vi "Mouse Move.vi"(7 "Map Model in":refnum<class "Map Model.lvclass">, 8 "error in (no error)":errorcluster, 10 "Position":T1, 11 "Pan in":refnum<class "Pan.lvclass">) -> (0 "error out":errorcluster, 3 "Pan out":refnum<class "Pan.lvclass">, 5 "Map Model out":refnum<class "Map Model.lvclass">)   [LabVIEW 2020, in "Map Model.lvlib" / "Pan.lvclass"]
uses:
  Pan.lvclass
  E:/Project/Labview-Projects/Completed projects/Map Editor/Models/Map Model/Tools/Tool/Tool.lvclass
  <vilib>/Utility/miscctls.llb/LVPoint32TypeDef.ctl
  Map Model/Map Model.lvclass
  Tool/Tool.lvclass/Tool.ctl
  Map Model/Map Model.lvclass/Map Model.ctl
  Undoable Tool/Undoable Tool.lvclass
  Tool/Tool.lvclass
  <vilib>/LabVIEW Icon API/lv_icon/lv_icon.lvlib
panel:
  # "NOTICE -- YOU MUST LEAVE THIS NOTICE IN PLACE.\n\nCopyright (c) 2017, LIANG LIU Shawn.Liu.cn@gmail.com\nAll rights reserved.\n\nRedistribution and use in source and binary forms, with or without modification, are permitted provided that the following conditions are met:\n-Redistributions of source code must retain the above copyright notice, this list of conditions and the following disclaimer.\n-Redistributions in binary form must reproduce the above copyright notice, this list of conditions and the following disclaimer in the documentation and/or other materials provided with the distribution.\n-Neither the name of the eLp nor the names of its contributors may be used to endorse or promote products derived from this software without specific prior written permission.\n\nTHIS SOFTWARE IS PROVIDED BY THE COPYRIGHT HOLDERS AND CONTRIBUTORS \"AS IS\" AND ANY EXPRESS OR IMPLIED WARRANTIES, INCLUDING, BUT NOT LIMITED TO, THE IMPLIED WARRANTIES OF MERCHANTABILITY AND FITNESS FOR A PARTICULAR PURPOSE ARE DISCLAIMED. IN NO EVENT SHALL THE COPYRIGHT HOLDER OR CONTRIBUTORS BE LIABLE FOR ANY DIRECT, INDIRECT, INCIDENTAL, SPECIAL, EXEMPLARY, OR CONSEQUENTIAL DAMAGES (INCLUDING, BUT NOT LIMITED TO, PROCUREMENT OF SUBSTITUTE GOODS OR SERVICES; LOSS OF USE, DATA, OR PROFITS; OR BUSINESS INTERRUPTION) HOWEVER CAUSED AND ON ANY THEORY OF LIABILITY, WHETHER IN CONTRACT, STRICT LIABILITY, OR TORT (INCLUDING NEGLIGENCE OR OTHERWISE) ARISING IN ANY WAY OUT OF THE USE OF THIS SOFTWARE, EVEN IF ADVISED OF THE POSSIBILITY OF SUCH DAMAGE."
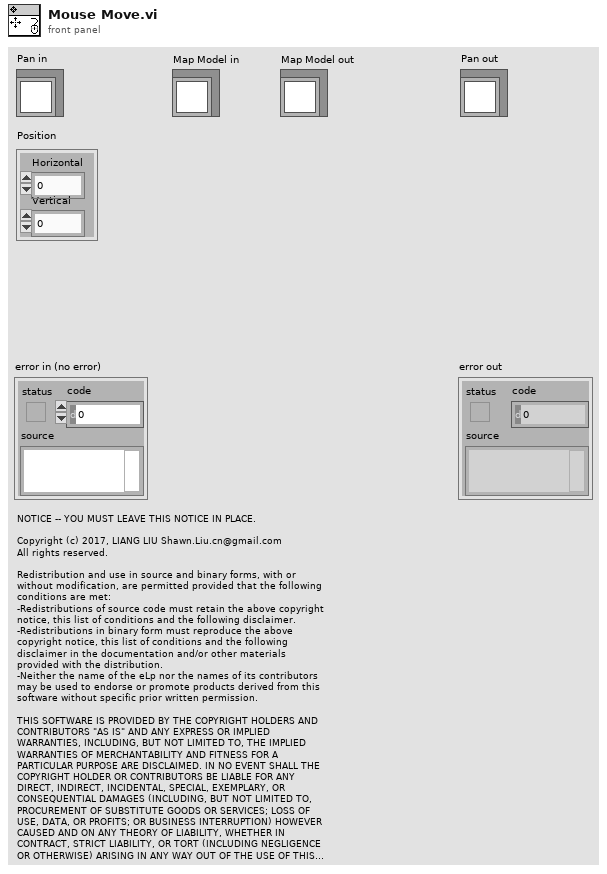
[diagram p1: front panel]
types:
  T1 = typedef "LVPoint32TypeDef.ctl" = cluster{"Horizontal":i32, "Vertical":i32}
  T2 = typedef "imagedata.ctl" = cluster{"image type":i32, "image depth":i32, "image":u8[], "mask":u8[], "colors":u32[], "Rectangle":cluster{"left":i16, "top":i16, "right":i16, "bottom":i16}}
  T3 = cluster{"left":i16, "top":i16, "right":i16, "bottom":i16}
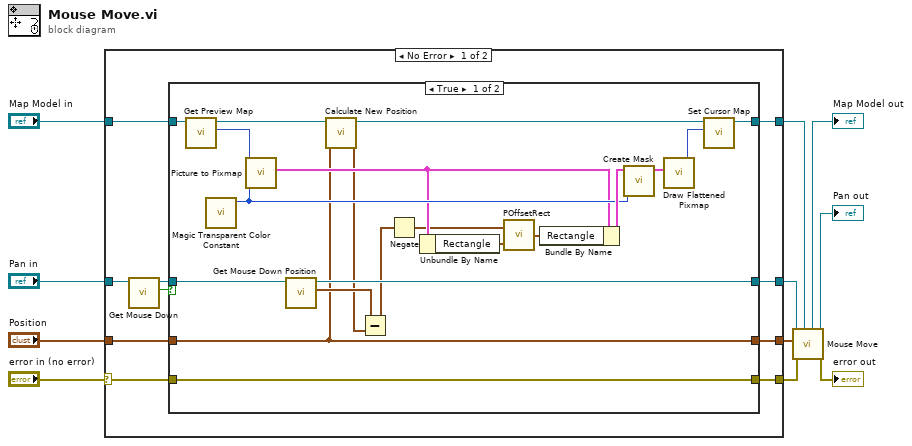
[diagram p0: block diagram]
diagram:
  n1 = case shown="No Error" "error in (no error)" {
    selector: "error in (no error)" -> [w19 w49]
    tunnel: "Map Model in" -> [w21 w48]
    tunnel: "Position" -> [w20 w46]
    tunnel: "Pan in" -> [w18 w47]
    tunnel: [w17 w46] -> w6
    tunnel: [w16 w48] -> w5
    tunnel: [w15 w47] -> w4
    tunnel: [w14 w49] -> w3
    frame No Error {
      n2 = call "Get Mouse Down.vi"("Tool in"=w18) -> ("Mouse Down"=w12:bool, "Tool out"=w13:refnum<class "Pan.lvclass">)  [unwired: 9 in]
      n3 = case shown="True" w12 {
        tunnel: w13 -> [w41 w45]
        tunnel: w21 -> [w39 w43]
        tunnel: [w22 w43] -> w16
        tunnel: [w40 w45] -> w15
        tunnel: w20 -> [w24 w42]
        tunnel: [w24 w42] -> w17
        tunnel: w19 -> [w38 w44]
        tunnel: [w38 w44] -> w14
        frame True {
          n4 = call "Get Preview Map.vi"("Map Model in"=w39) -> ("Preview Map"=w27:picture, "Map Model out"=w28:refnum<class "Map Model.lvclass">)  [unwired: 9 in]
          n5 = call <vilib>:"Magic Transparent Color Constant.vi"() -> ("Magic transparent color constant"=w31:u32)  [unwired: 11 in]
          n6 = call <vilib>:"Picture to Pixmap.vi"("Background Color"=w31, "picture"=w27) -> ("image data"=w30:T2)  [unwired: 8 in, 1 out]
          n7 = call "Get Mouse Down Position.vi"("Tool in"=w41) -> ("Mouse Down Position"=w34:T1, "Tool out"=w40:refnum<class "Pan.lvclass">)  [unwired: 9 in]
          n8 = call "Calculate New Position.vi"("Position in"=w24, "Map Model in"=w28) -> ("Position out"=w23:T1, "Map Model out"=w25:refnum<class "Map Model.lvclass">)  [unwired: 8 in]
          n9 = Subtract(x=w34, y=w23) -> (x-y=w37:T1)
          n10 = Negate(x=w37) -> (-x=w26:T1)
          n11 = Unbundle By Name(w30) -> ("Rectangle"=w36:T3)
          n12 = call <vilib>:"POffsetRect.vi"("rect"=w36, "point"=w26) -> ("offset rect"=w35:T3)
          n13 = Bundle By Name(cluster=w30, "Rectangle"=w35) -> (w32:T2)
          n14 = call <vilib>:"Create Mask.vi"("Mask Color (Black)"=w31, "image data"=w32) -> ("image data"=w33:T2)  [unwired: 9 in]
          n15 = call <vilib>:"Draw Flattened Pixmap.vi"("image data"=w33) -> ("new picture"=w29:picture)  [unwired: 8 in]
          n16 = call "Set Cursor Map.vi"("Cursor Map"=w29, "Map Model in"=w25) -> ("Map Model out"=w22:refnum<class "Map Model.lvclass">)  [unwired: 9 in]
        }
        frame False {
        }
      }
    }
    frame Error {
    }
  }
  n17 = call-parent "Mouse Move.vi"("Map Model in"=w5, "error in (no error)"=w3, "Position"=w6, "Tool in"=w4) -> ("error out"=→"error out":errorcluster, "Tool out"=→"Pan out":refnum<class "Pan.lvclass">, "Map Model out"=→"Map Model out":refnum<class "Map Model.lvclass">)  [unwired: 5 in]
